vi "Load Device Config.vi"(8 "Error In":errorcluster, 11 "LINX Device Config":T1) -> (0 "Error Out":errorcluster, 3 "LINX Device Config":T1)   [LabVIEW 2011, in "LVH-LINX.lvlib" / "Device.lvlib"]
uses:
  Device.lvlib
  Type Defs/LINX Device Config.ctl
  Type Defs/Interface.ctl
  Type Defs/TCP Config.ctl
  Type Defs/Channels.ctl
  LVH-LINX.lvlib
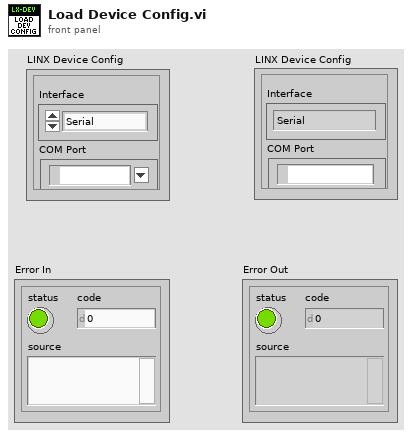
[diagram p1: front panel]
types:
  T1 = typedef "LVH-LINX.lvlib/Device.lvlib/LINX Device Config.ctl" = cluster{"Interface":T2, "COM Port":refnum<visa-resource-name>, "TCP Configuration":T3, "Device Family":u8, "Device ID":u8, "Device Name":string, "TCP Ref":refnum<k5>, "Channels":T4}
  T2 = typedef "LVH-LINX.lvlib/Interface.ctl" = enum16{"Serial", "TCP"}
  T3 = typedef "LVH-LINX.lvlib/Device.lvlib/TCP Config.ctl" = cluster{"IP Address":string, "Port":u16}
  T4 = typedef "LVH-LINX.lvlib/Channels.ctl" = cluster{"DI":u8[], "DO":u8[], "AI":u8[], "AO":u8[], "PWM":u8[], "QE":u8[], "UART":u8[], "I2C 2":u8[], "SPI":u8[], "CAN":u8[], "Servo":u8[], "AI Ref (V)":dbl, "AO Ref (V)":dbl, "AO Resolution (Bits)":u8}
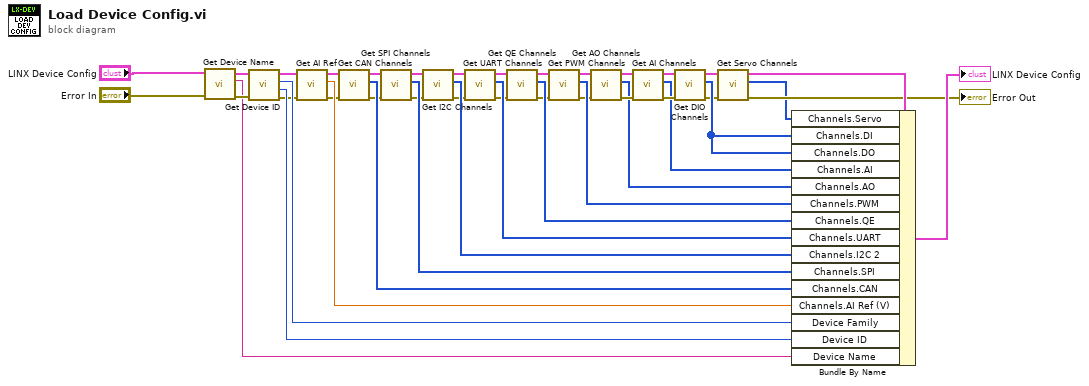
[diagram p0: block diagram]
diagram:
  n1 = call "Get Device Name.vi"("Error In"="Error In", "LINX Device Config"="LINX Device Config") -> ("Error Out"=w10:errorcluster, "Device Name"=w6:string, "LINX Device Config"=w9:T1)  [unwired: 7 in]
  n2 = call "Get Device ID.vi"("Error In"=w10, "LINX Device Config"=w9) -> ("Error Out"=w20:errorcluster, "Device ID"=w36:u8, "Device Family"=w35:u8, "LINX Device Config"=w19:T1)  [unwired: 6 in]
  n3 = call "Get AI Ref.vi"("Error In"=w20, "LINX Device Config"=w19) -> ("Error Out"=w21:errorcluster, "AI Ref"=w34:dbl, "LINX Device Config"=w18:T1)  [unwired: 7 in]
  n4 = call "Get CAN Channels.vi"("Error In"=w21, "LINX Device Config"=w18) -> ("Error Out"=w22:errorcluster, "CAN Channels"=w33:u8[], "LINX Device Config"=w17:T1)  [unwired: 6 in, 1 out]
  n5 = call "Get SPI Channels.vi"("Error In"=w22, "LINX Device Config"=w17) -> ("Error Out"=w23:errorcluster, "SPI Channels"=w32:u8[], "LINX Device Config"=w16:T1)  [unwired: 6 in, 1 out]
  n6 = call "Get I2C Channels.vi"("Error In"=w23, "LINX Device Config"=w16) -> ("Error Out"=w24:errorcluster, "I2C Channels"=w31:u8[], "LINX Device Config"=w15:T1)  [unwired: 6 in, 1 out]
  n7 = call "Get UART Channels.vi"("Error In"=w24, "LINX Device Config"=w15) -> ("Error Out"=w25:errorcluster, "UART Channels"=w30:u8[], "LINX Device Config"=w14:T1)  [unwired: 6 in, 1 out]
  n8 = call "Get QE Channels.vi"("Error In"=w25, "LINX Device Config"=w14) -> ("Error Out"=w26:errorcluster, "QE Channels"=w29:u8[], "LINX Device Config"=w13:T1)  [unwired: 6 in, 1 out]
  n9 = call "Get PWM Channels.vi"("Error In"=w26, "LINX Device Config"=w13) -> ("Error Out"=w27:errorcluster, "PWM Channels"=w28:u8[], "LINX Device Config"=w12:T1)  [unwired: 6 in, 1 out]
  n10 = call "Get AO Channels.vi"("Error In"=w27, "LINX Device Config"=w12) -> ("Error Out"=w43:errorcluster, "AI Channels"=w37:u8[], "LINX Device Config"=w41:T1)  [unwired: 6 in, 1 out]
  n11 = call "Get AI Channels.vi"("Error In"=w43, "LINX Device Config"=w41) -> ("Error Out"=w42:errorcluster, "AI Channels"=w38:u8[], "LINX Device Config"=w40:T1)  [unwired: 6 in, 1 out]
  n12 = call "Get DIO Channels.vi"("Error In"=w42, "LINX Device Config"=w40) -> ("Error Out"=w3:errorcluster, "DIO Channels"=w39:u8[], "LINX Device Config"=w5:T1)  [unwired: 6 in, 1 out]
  n13 = call "Get Servo Channels.vi"("Error In"=w3, "LINX Device Config"=w5) -> ("Error Out"=→"Error Out":errorcluster, "Servo Channels"=w1:u8[], "LINX Device Config"=w4:T1)  [unwired: 6 in, 1 out]
  n14 = Bundle By Name(cluster=w4, "Channels.Servo"=w1, "Channels.DI"=w39, "Channels.DO"=w39, "Channels.AI"=w38, "Channels.AO"=w37, "Channels.PWM"=w28, "Channels.QE"=w29, "Channels.UART"=w30, "Channels.I2C 2"=w31, "Channels.SPI"=w32, "Channels.CAN"=w33, "Channels.AI Ref (V)"=w34, "Device Family"=w35, "Device ID"=w36, "Device Name"=w6) -> (→"LINX Device Config":T1)
